vi "AlliGator Get Frame Number in .ptu File.vi"(8 "error in (no error)":errorcluster, 11 "File Path":path) -> (0 "error out":errorcluster, 3 "# Frames":i32)   [LabVIEW 2021, in "AlliGator Files.lvlib"]
doc: "Hack to figure out the number of \"frames\"in a .ptu files generaetd by the Leica FLIM confocal microscope (basically reading the entire file)."
uses:
  AlliGator Files.lvlib
  AlliGator FLI Image Stack Action.ctl
  AlliGator Variables List.ctl
  Variant/Variant to Data/Variant to I32.vi
  AlliGator HDF5.lvlib
  AlliGator Globals, Variables & Constants.lvlib
  Variant/Variant to Data/Variant to Data.lvlib
panel:
  # "see the AlliGator License on the block diagram (Ctrl+E or Window:Show Block Diagram)"
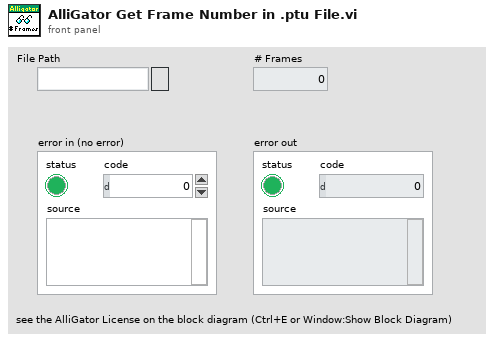
[diagram p1: front panel]
types:
  T1 = typedef "AlliGator Globals, Variables & Constants.lvlib/AlliGator Variables List.ctl" = enum16{"---- GUI ----", "Initialization Status", "State Indicators Refnum", "Original AlliGator Menu Items", "Current Action Loop State", "Script in progress", "Playback", "Loop Playback", "Search ROI Used", "Search ROI", "Decay Graph Max Legend Size", "Intensity Graph Max Legend Size", "Decay Statistics Graph Max Legend Size", "Phasor Graph Max Legend Size", "Phasor Ratio Graph Max Legend Size", "Lifetime Graph Max Legend Size", "---- Files ----", "Export Dataset Frames as Individual Files", "Show Batch Export Help Balloons", "Frames in Dataset", "ptu File Frame Start Indices", "Current Frame in Dataset", "Current Frame Timestamp", "------ Python Plugins ------", "Python Plugins Information", "Python Session", "Valid Python Session?", "---- Source Image ----", "Dataset Loaded", "Dataset Metadata", "Dataset Channel", "Dataset Data Description", "Background Dataset Metadata", "Background Dataset Channel", "Background Dataset Data Description", "Background File Subtraction", "Background File Path", "Background File Pile-up Correction", "Background File Pixel Well Capacity", "Background File Scaling Factor", "Source Image ROIs", "Current Source Image ROI", "Source Image ROI Event Refnum", "X_Source Image Display Range", "X_Source Image Palette Information", "Source Image Palette List", "Source Image Scale", "Current Dataset Load Settings", "Source Image:ROI Overlay Color", "---- Image Profile Window ----", "Image Profile:Overlay ROI in Source Image", "Image Profile Window Event Refnum", "Image Profile:IntensityType", "Image Profile:Intensity Average Type", "Image Profile:Intensity-weighted SDV", "Image Profile:Box Profile Type", "Image Profile Window Open", "Image Profile:Plotted Fit Parameter", "X_Type of Displayed Image", "X_Time Gate Slider", "Dataset Path", "Source Image Overlay to Erase", "Is Displayed Image Accumulated", "White Light Image Modified", "Mask Image Modified", "Macrotime Gate Separation", "------ Phasor Graph -------", "Phasor Graph:Show Line", "---- Phasor Plot ---", "Phasor Plot Parameters Changed", "FLI Dataset Modified since last Phasor Plot Calculation", "Phasor Harmonics Data", "Selected Phasor Harmonics", "Phasor Harmonic Manager Event Refnum", "Phasor Plot ROIs", "Current Phasor Plot ROI", "Phasor Plot ROI Event Refnum", "Phasor Plot Image Reference Points", "Phasor Plot Computed", "Phasor Plot Palette Information", "Phasor Plot Palette List", "Phasor Ratio Palette Information", "Phasor Ratio Palette List", "Phasor Image Scale", "Phasor Plot Image Overlay to Erase", "Phasor Plot Image Elements to Update", "Current Phasor Plot Calculation Parameters", "Current Phasor Calibration Options", "Reset Cumulated Phasor Plot", "Phasor Ratio Reference 1", "Phasor Ratio Lifetime Reference 1", "Phasor Ratio Reference 1 Frequency", "Phasor Ratio Reference 2", "Phasor Ratio Lifetime Reference 2", "Phasor Ratio Reference 2 Frequency", "---- Decay Analysis ----", "Number of Selected Decays to Fit", "LS Fit Results", "LAR Fit Results", "BS Fit Results", "Last Decay Max - Min", "Best Fit Parameters", "Best Fit Parameter Names", "Actual Size X", "Actual Size Y", "Binning X", "Binning Y", "Actual # Gates", "Dataset Number", "Gates to...", "Gates Skipped", "Gates to keep", "Gate Step", "Gate Separation", "Reversed Gates", "Pile-up Correction", "Pixel Well Capacity", "Background Subtracted", "Background Subtraction Method", "Background Definition Range", "Background File (deprecated)", "Number of Dataset Accumulated", "Array of Accumulated Dataset Paths", "Do Averaged Datasets", "Destination File Path", "Process Plot Target", "Use 1/D as Phasor Frequency", "---- Decay Fit Parameter Map -----", "Decay Fit Parameter Map Palette Information", "Decay Fit Parameter Map Palette List", "Local Decay Graph Window Event Refnum", "------- Local Decay Window ---------", "Use normalized IRF for convolution", "----- Miscellaneous ----", "Skippable Dialog Windows Status"}
  T2 = typedef "AlliGator HDF5.lvlib/AlliGator FLI Image Stack Action.ctl" = enum16{"Init", "Get Image", "Close"}
  T3 = typedef "PicoQuant.lvlib/Extended PicoQuant Data File Information.ctl" = cluster{"File Path":path, "Data offset (in bytes)":i64, "PicoQuant Data File Information":T4, "User defined # Gates":i64, "User defined Bin Size (s)":dbl, "p (# native bins per user bin)":dbl}
  T4 = typedef "PTU Files.lvlib/PicoQuant Data File Information.ctl" = cluster{"PQ File Information":T5, "PQ Software Information":T6, "PQ Remote Request Information":T7, "PQ Hardware Information":T8, "PQ Measurement Information":T13, "PQ Image Information":T14, "PQ TT Results Format Information":T15, "PQ Measurement Results":T16}
  T5 = typedef "PTU Files.lvlib/PicoQuant File Information.ctl" = cluster{"GUID":string, "Assured Content":string, "Measurement Mode":i64, "Measurement SubMode":i64, "Comment":string, "Creation Time":string}
  T6 = typedef "PTU Files.lvlib/PicoQuant Software Information.ctl" = cluster{"Content Version":string, "Name":string, "Version":string, "# Modules":i64, "Module Names":string[], "Module Versions":string[], "SVN Build":i64}
  T7 = typedef "PTU Files.lvlib/PicoQuant Remote Request Information.ctl" = cluster{"Started by Remote Interface":bool, "Measurement Type":i64, "# Pixel X":i64, "# Pixel Y":i64, "Record Version":i64, "Scanning Pattern":i64, "Scanning Resolution (m/px)":dbl, "Comment":string, "File Name":string, "Group Name":string}
  T8 = typedef "PTU Files.lvlib/PicoQuant Hardware Information.ctl" = cluster{"Input Channels":T9, "Markers":T10, "Modules":T11, "Router Channels":T12}
  T9 = typedef "PTU Files.lvlib/PicoQuant Input Channels.ctl" = cluster{"# Input Channels":i64, "CFD Levels (mV)":i64[], "CFD Zero Crossings (mV)":i64[], "CFD Channel Enabled":bool[], "Module Indices":i64[], "Offsets (ps)":i64[], "Td Codes":i64[], "Trigger Edges":i64[], "Trigger Levels (mV)":i64[]}
  T10 = typedef "PTU Files.lvlib/PicoQuant Markers.ctl" = cluster{"# Markers":i64, "Markers Enabled":bool[], "Holdoff (ns)":i64, "Rising Edges":bool[]}
  T11 = typedef "PTU Files.lvlib/PicoQuant Modules.ctl" = cluster{"# Modules":i64, "Type Codes":i64[], "Version Codes":i64[]}
  T12 = typedef "PTU Files.lvlib/PicoQuant Router Channels.ctl" = cluster{"# Router Channels":i64, "CFD Levels (mV)":i64[], "CFD Present":bool[], "CFD Zero Crossings (mV)":i64[], "Input Levels (mV)":i64[], "Input Types":i64[], "Offsets (ps)":i64[], "Rising Edges":bool[], "Router Enabled":bool, "Router Model Code":i64, "Router Version":string, "Sync CFD Level (mV)":i64, "Sync CFD Zero Crossing (mV)":i64, "Sync Divider":i64, "Sync Offset (ps)":i64, "Sync Trigger Edge":i64, "Sync Trigger Level (mV)":i64, "Trigger Out On":bool, "Trigger Out Period (s)":dbl, "Base Resolution (s)":dbl, "External Devices":i64, "External Reference Clock":bool, "Features":u64, "Part Number":string, "Serial Number (string)":string, "Serial Number":i64, "Timing Mode":i64, "Hardware Type":string, "Hardware Version":string}
  T13 = typedef "PTU Files.lvlib/PicoQuant Measurement Information.ctl" = cluster{"Acquisition Time (ms)":i64, "Binning Factor":i64, "Global Resolution (s)":dbl, "Invalid Sync":bool, "Offset (ns)":u64, "# Curve Parameters":u64, "Devices":string[], "Names":string[], "Start Values":dbl[], "Steps":dbl[], "Stop Values":dbl[], "Tag Names":string[], "Units":string[], "Resolution (s)":dbl, "Restart":bool, "Stop At":u64, "Stop on Over f1":bool}
  T14 = typedef "PTU Files.lvlib/PicoQuant Image Information.ctl" = cluster{"Hardware Acceleration":i64, "Bidirectional":bool, "Dimensions":i64, "Frame Marker":i64, "Scanner Identity":i64, "Learning Time (s)":i64, "Line Frequency":dbl, "Line Start Marker":i64, "Line Stop Marker":i64, "Max Frames":i64, "Objective Name":string, "Pixel Resolution (um)":dbl, "# Pixels X":i64, "# Pixels Y":i64, "Preview Pixels/Line":i64, "Scan Direction":i64, "Sinusoidal Correction":i64, "Time per Line (ms)":dbl, "Time per Pixel (ms)":i64, "Velocity":i64, "X0 (um)":dbl, "X1 (um)":dbl, "X Calibration Offset (V)":dbl, "X Calibration (m/V)":dbl, "Y0 (um)":dbl, "Y1 (um)":dbl, "Y Calibration Offset (V)":dbl, "Y Calibration (m/V)":dbl, "Z0 (um)":dbl, "Z1 (um)":dbl, "Z Calibration Offset (V)":dbl, "Z  Calibration (m/V)":dbl}
  T15 = typedef "PTU Files.lvlib/PicoQuant Results Format.ctl" = cluster{"Bits per Record":i64, "Channel Mask":i64, "Channel Shift ":i64, "DTime Mask":i64, "DTime Shift":i64, "Marker Mask":i64, "Marker Shift":i64, "NSync Mask":i64, "NSync Shift":i64, "Special Mask":i64, "TTTR Record Type":i64, "Wrap Around":i64}
  T16 = typedef "PTU Files.lvlib/PicoQuant Measurement Results.ctl" = cluster{"Stop Reason":i64, "Input Rates (cps)":i64[], "Warning Flags":u64, "# Records":i64, "Stop After (ms)":i64, "Sync Rate (cps)":i64}
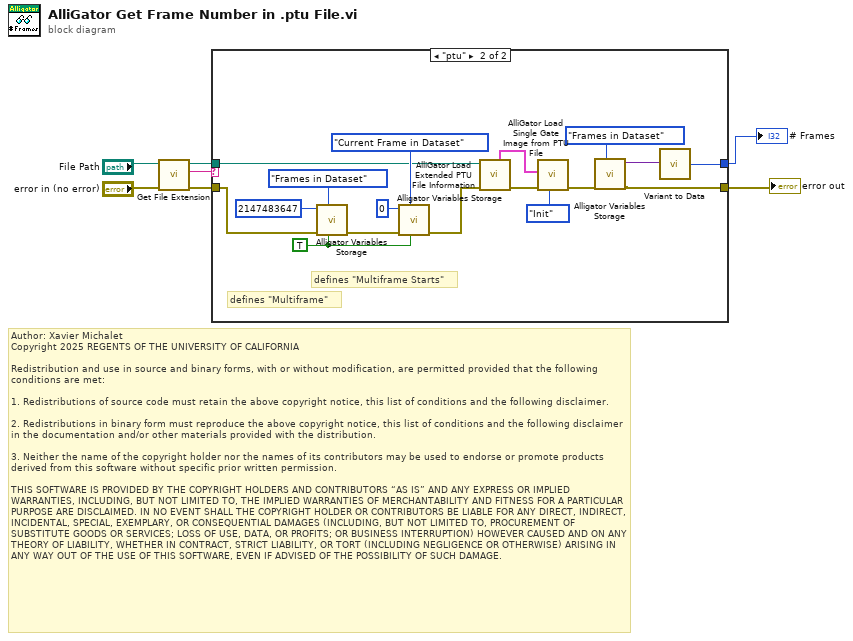
[diagram p0: block diagram]
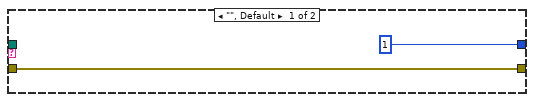
[diagram p2: hidden frame]
diagram:
  # "Author: Xavier Michalet\nCopyright 2025 REGENTS OF THE UNIVERSITY OF CALIFORNIA\n\nRedistribution and use in source and binary forms, with or without modification, are permitted provided that the following conditions are met:\n\n1. Redistributions of source code must retain the above copyright notice, this list of conditions and the following disclaimer.\n\n2. Redistributions in binary form must reproduce the above copyright notice, this list of conditions and the following disclaimer in the documentation and/or other materials provided with the distribution.\n\n3. Neither the name of the copyright holder nor the names of its contributors may be used to endorse or promote products derived from this software without specific prior written permission.\n\nTHIS SOFTWARE IS PROVIDED BY THE COPYRIGHT HOLDERS AND CONTRIBUTORS “AS IS” AND ANY EXPRESS OR IMPLIED WARRANTIES, INCLUDING, BUT NOT LIMITED TO, THE IMPLIED WARRANTIES OF MERCHANTABILITY AND FITNESS FOR A PARTICULAR PURPOSE ARE DISCLAIMED. IN NO EVENT SHALL THE COPYRIGHT HOLDER OR CONTRIBUTORS BE LIABLE FOR ANY DIRECT, INDIRECT, INCIDENTAL, SPECIAL, EXEMPLARY, OR CONSEQUENTIAL DAMAGES (INCLUDING, BUT NOT LIMITED TO, PROCUREMENT OF SUBSTITUTE GOODS OR SERVICES; LOSS OF USE, DATA, OR PROFITS; OR BUSINESS INTERRUPTION) HOWEVER CAUSED AND ON ANY THEORY OF LIABILITY, WHETHER IN CONTRACT, STRICT LIABILITY, OR TORT (INCLUDING NEGLIGENCE OR OTHERWISE) ARISING IN ANY WAY OUT OF THE USE OF THIS SOFTWARE, EVEN IF ADVISED OF THE POSSIBILITY OF SUCH DAMAGE."
  n1 = call <vilib>:"Get File Extension.vi"("error in (no error)"="error in (no error)", "file"="File Path") -> ("error out"=w4:errorcluster, "lowercase file extension"=w6:string, "dup file"=w3:path)  [unwired: 5 in, 2 out]
  n2 = case shown="\"ptu\"" w6 {
    tunnel: w4 -> [w8 w15]
    tunnel: w3 -> [_ w13]
    tunnel: [1 ("# Frames") w20] -> w1
    tunnel: [w8 w23] -> w2
    frame "", Default {
    }
    frame "ptu" {
      w11 = TRUE ("Get(F)/Set")
      # "defines \"Multiframe Starts\""
      # "defines \"Multiframe\""
      n3 = call "Alligator Variables Storage.vi"("Get(F)/Set"=w11, "AlliGator Variable"=AlliGator_Variables_List."Frames in Dataset" ("Alligator Variable"), "Error In"=w15, "Data in"=2147483647 ("# Frames")) -> ("Error Out"=w19:errorcluster)  [unwired: 5 in, 2 out]
      n4 = call "Alligator Variables Storage.vi"("Get(F)/Set"=w11, "AlliGator Variable"=AlliGator_Variables_List."Current Frame in Dataset" ("Alligator Variable"), "Error In"=w19, "Data in"=0 ("# Frames")) -> ("Error Out"=w14:errorcluster)  [unwired: 5 in, 2 out]
      n5 = call "AlliGator Load Extended PTU File Information.vi"("Error In"=w14, "File Path"=w13) -> ("Error Out"=w26:errorcluster, "Extended ptu File Information"=w10:T3)  [unwired: 3 in, 5 out]
      n6 = call "AlliGator Load Single Gate Image from PTU File.vi"("Action"=AlliGator_FLI_Image_Stack_Action."Init", "error in (no error)"=w26, "File Info"=w10) -> ("error out"=w24:errorcluster)  [unwired: 6 in, 2 out]
      n7 = call "Alligator Variables Storage.vi"("AlliGator Variable"=AlliGator_Variables_List."Frames in Dataset" ("Alligator Variable"), "Error In"=w24) -> ("Error Out"=w23:errorcluster, "Data out"=w21:variant)  [unwired: 7 in, 1 out]
      n8 = call-poly "Variant to Data.vi"("Variant"=w21) -> ("Value"=w20:i32)  [unwired: 8 in]
    }
  }
  "# Frames" <- w1
  "error out" <- w2
